vi "Drive_Loop_Cheesey_Drive.vi"(9 "Wheel":dbl, 10 "Throttle":dbl, 11 "Drive Loop Cluster":T1) -> ()   [LabVIEW 2016]
doc: "Help writen by FRC Team 836 - The RoboBees\n\nVI places robot in manual drive mode with speed and steering commands.\n\nThis VI takes throttle and steering commands and writes them with the \"Manual\" mode command to the Drive Command RT FIFO in the\nDrive Loop Cluster.\n\nThe RT FIFO has to be initialized using the \"Drive_Loop_Initialize_w_Help\" VI."
uses:
  <userlib>/836-libraries/Drive/Drive_Code/Drive_Code_Support/Drive_Code_Bundle.ctl
  <userlib>/836-libraries/Drive/Drive_Code/Drive_Code_Support/Sensor_Cluster.ctl
  <userlib>/836-libraries/Drive/Drive_Code/Drive_Code_Support/Camera_Cluster.ctl
  <userlib>/836-libraries/Drive/Drive_Code/Drive_Code_Support/Drive_Code_Notifier.ctl
  <userlib>/836-libraries/Drive/Drive_Code/Drive_Code_Support/Drive_Code_Command.ctl
  <userlib>/836-libraries/Drive/Drive_Code/Logging_Data.ctl
  <userlib>/836-libraries/Drive/Drive_Code/Drive_Code_Support/Drive_Code_PID_Bundle.ctl
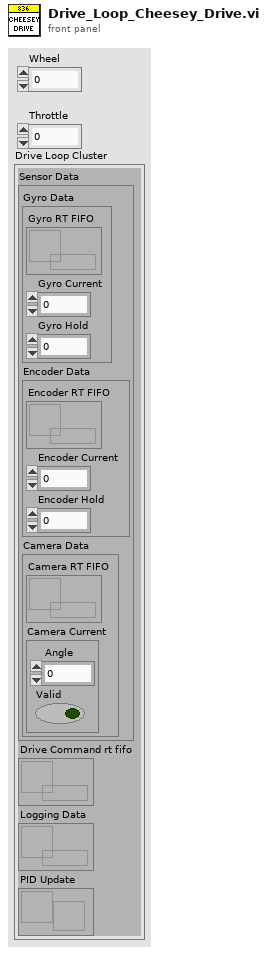
[diagram p1: front panel]
types:
  T1 = typedef "Drive_Code_Bundle.ctl" = cluster{"Sensor Data":T2, "Drive Command rt fifo":refnum<k33>, "Logging Data":refnum<k33>, "PID Update":refnum<notifier>}
  T2 = typedef "Sensor_Cluster.ctl" = cluster{"Gyro Data":cluster{"Gyro RT FIFO":refnum<k33>, "Gyro Current":dbl, "Gyro Hold":dbl}, "Encoder Data":cluster{"Encoder RT FIFO":refnum<k33>, "Encoder Current":dbl, "Encoder Hold":dbl}, "Camera Data":cluster{"Camera RT FIFO":refnum<k33>, "Camera Current":T3}}
  T3 = typedef "Camera_Cluster.ctl" = cluster{" Angle":dbl, "Valid":bool}
  T4 = typedef "Drive_Code_Command.ctl" = enum16{"Do Nothing", "Manual", "Drive Continuous", "Turn", "Drive Distance", "Hold Position", "Hold Yaw", "Follow Camera", "Turn to Camera"}
  T5 = typedef "Drive_Code_Notifier.ctl" = cluster{"Command":T4, "Parameter A":dbl, "Parameter B":dbl, "Parameter C":dbl, "Absolute?":bool}
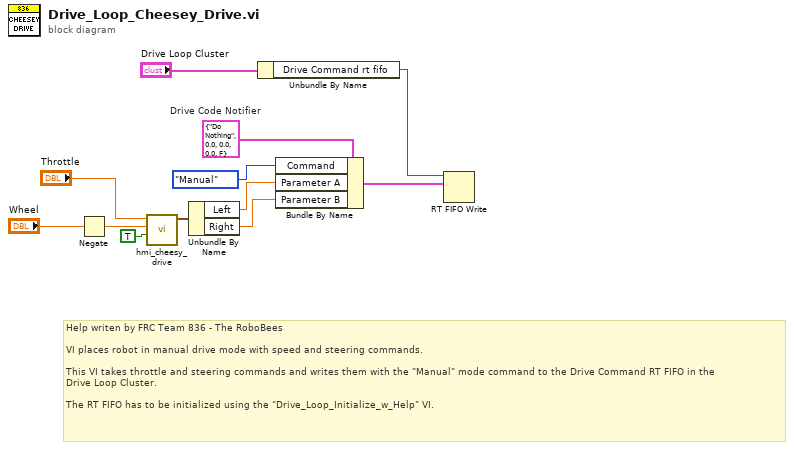
[diagram p0: block diagram]
diagram:
  w1 = T5 {"Command"=enum."Do Nothing", "Parameter A"=0.0, "Parameter B"=0.0, "Parameter C"=0.0, "Absolute?"=FALSE}  # Drive Code Notifier
  # "Help writen by FRC Team 836 - The RoboBees\n\nVI places robot in manual drive mode with speed and steering commands.\n\nThis VI takes throttle and steering commands and writes them with the \"Manual\" mode command to the Drive Command RT FIFO in the\nDrive Loop Cluster.\n\nThe RT FIFO has to be initialized using the \"Drive_Loop_Initialize_w_Help\" VI."
  n1 = Negate(x="Wheel") -> (-x=w6:dbl)
  n2 = call <userlib>:"hmi_cheesy_drive.vi"("Quick Turn"=TRUE, "Wheel"=w6, "Throttle"="Throttle") -> ("Drive Data"=w7:cluster{"Left":dbl, "Right":dbl})  [unwired: 8 in]
  n3 = Unbundle By Name(w7) -> ("Left"=w8:dbl, "Right"=w9:dbl)
  n4 = Unbundle By Name("Drive Loop Cluster") -> ("Drive Command rt fifo"=w12:refnum<k33>)
  n5 = Bundle By Name(cluster=w1, "Command"=Drive_Code_Command."Manual", "Parameter A"=w8, "Parameter B"=w9) -> (w11:T5)
  n6 = RT FIFO Write(0:w12, 1:w11) -> ()  [unwired: 3 in, 4 out]
